vi "ReadSubVI.vi"(8 "error in (no error)":errorcluster, 11 "reference":refnum<visa-resource-name>) -> (0 "error out":errorcluster, 1 "number":dbl, 2 "before substring":string, 3 "VISA resource name out":refnum<visa-resource-name>, 4 "Bytes at port":u32, 5 "read buffer":string)   [LabVIEW 2018]
panel:
  out "after substring":string
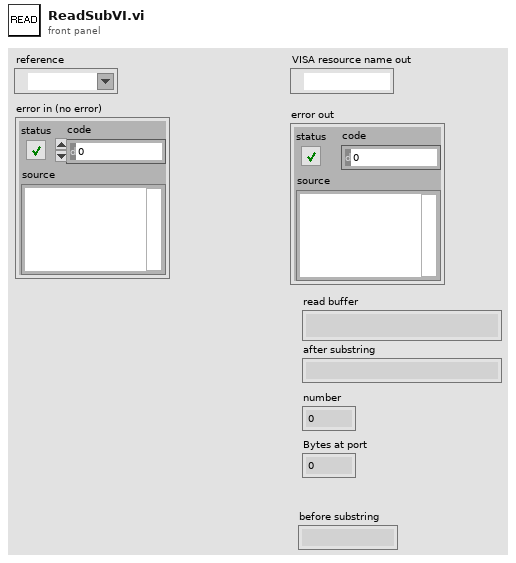
[diagram p1: front panel]
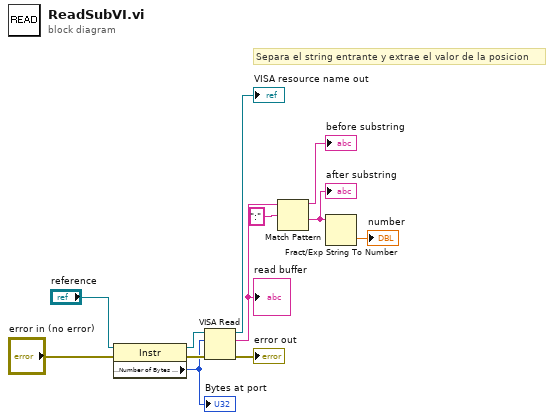
[diagram p0: block diagram]
diagram:
  # "Separa el string entrante y extrae el valor de la posicion"
  n1 = property class="Instr"(reference="reference", error in="error in (no error)") -> (reference out=w12:refnum<visa-resource-name>, error out=w8:errorcluster, "Serial Settings:Number of Bytes at Serial Port"=w3:u32)
  "Bytes at port" <- w3
  n2 = VISA Read(VISA resource name=w12, byte count=w3, error in (no error)=w8) -> (VISA resource name out=→"VISA resource name out":refnum<visa-resource-name>, read buffer=w11:string, error out=→"error out":errorcluster)  [unwired: 1 out]
  "read buffer" <- w11
  n3 = Match Pattern(string=w11, regular expression=":") -> (before substring=→"before substring":string, after substring=w9:string)  [unwired: 1 in, 2 out]
  "after substring" <- w9
  n4 = Fract/Exp String To Number(string=w9) -> (number=→"number":dbl)  [unwired: 3 in, 1 out]
